vi "configure.vi"(8 "error in (no error)":errorcluster, 9 "PGA Gain":u8 max=7, 10 "ADC Configuration":string, 11 "ILC in":refnum<class "ILC.lvclass">) -> (0 "error out":errorcluster, 3 "ILC out":refnum<class "ILC.lvclass">)   [LabVIEW 2015, in "ILCCommon.lvlib" / "ILC.lvclass"]
uses:
  <userlib>/Common/ILC/ILC/ILC.lvclass
  <userlib>/Common/ILC/ILC/ILC.lvclass/ILC.ctl
  <userlib>/Common/SerialProtocols/SerialCommunicator/SerialCommunicator.lvclass
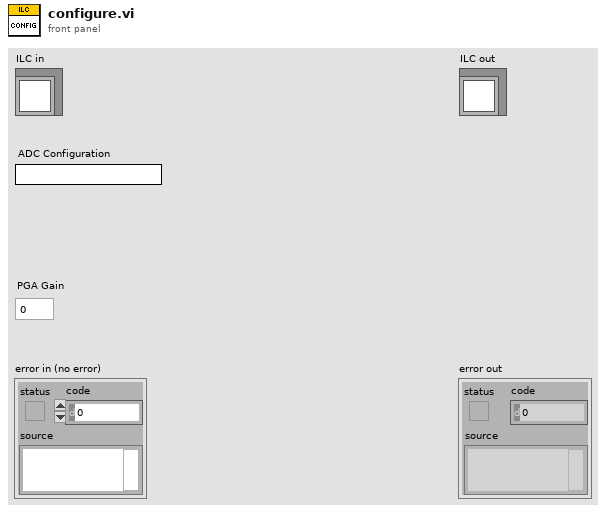
[diagram p1: front panel]
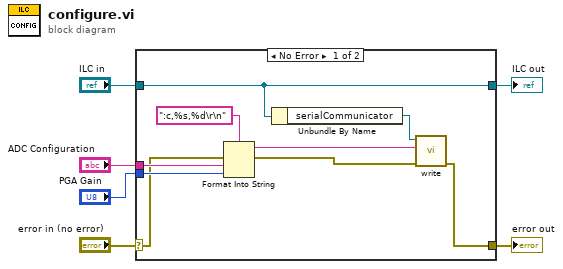
[diagram p0: block diagram]
diagram:
  n1 = case shown="No Error" "error in (no error)" {
    selector: "error in (no error)" -> [w8 w17]
    tunnel: [w7 w17] -> w5
    tunnel: [w15 w16] -> w3
    tunnel: "ILC in" -> [w15 w16]
    tunnel: "ADC Configuration" -> [w13 _]
    tunnel: "PGA Gain" -> [w12 _]
    frame No Error {
      n2 = Format Into String(format string=":c,%s,%d\r\n", error in=w8, w13, w12) -> (resulting string=w10:string, error out=w9:errorcluster)  [unwired: 1 in]
      n3 = Unbundle By Name(w15) -> ("serialCommunicator"=w11:refnum<class "SerialCommunicator.lvclass">)
      n4 = call-dynamic "write.vi"("error in (no error)"=w9, "writeString"=w10, "SerialCommunicator in"=w11) -> ("error out"=w7:errorcluster)  [unwired: 7 in, 1 out]
    }
    frame Error {
    }
  }
  "error out" <- w5
  "ILC out" <- w3
